vi "Actor Core.vi"(8 "error in":errorcluster, 11 "PS in":refnum<class "Power Supply.lvclass">) -> (0 "error out":errorcluster, 3 "Actor out":refnum<class "Actor.lvclass">)   [LabVIEW 2019, in "Power Supply.lvlib" / "Power Supply.lvclass"]
doc: "The user interface for this panel.\n\n----\nPlease see the following web address for additional documentation and tutorial information:\nhttp://www.mooregoodideas.com/mgi-panel-manager/\n\nAuthor: Derek Trepanier\n\nCopyright (c) 2018, Moore Good Ideas, Inc.\n\nAll rights reserved.\n\nRedistribution and use in source and binary forms, with or without modification, are permitted provided that the following conditions are met:\n\n * Redistributions of source code must retain the above copyright notice, this list of conditions and the following disclaimer.\n * Redistributions in binary form must reproduce the above copyright notice, this list of conditions and the following disclaimer in the documentation and/or other materials provided with the distribution.\n * Neither the name of Moore Good Ideas, Inc. nor the names of its contributors may be used to endorse or promote products derived from this software without specific prior written permission.\n\nTHIS SOFTWARE IS PROVIDED BY THE COPYRIGHT HOLDERS AND CONTRIBUTORS \"AS IS\" AND ANY EXPRESS OR IMPLIED WARRANTIES, INCLUDING, BUT NOT LIMITED TO, THE IMPLIED WARRANTIES OF MERCHANTABILITY AND FITNESS FOR A PARTICULAR PURPOSE ARE DISCLAIMED. IN NO EVENT SHALL THE COPYRIGHT OWNER OR CONTRIBUTORS BE LIABLE FOR ANY DIRECT, INDIRECT, INCIDENTAL, SPECIAL, EXEMPLARY, OR CONSEQUENTIAL DAMAGES (INCLUDING, BUT NOT LIMITED TO, PROCUREMENT OF SUBSTITUTE GOODS OR SERVICES; LOSS OF USE, DATA, OR PROFITS; OR BUSINESS INTERRUPTION) HOWEVER CAUSED AND ON ANY THEORY OF LIABILITY, WHETHER IN CONTRACT, STRICT LIABILITY, OR TORT (INCLUDING NEGLIGENCE OR OTHERWISE) ARISING IN ANY WAY OUT OF THE USE OF THIS SOFTWARE, EVEN IF ADVISED OF THE POSSIBILITY OF SUCH DAMAGE."
uses:
  Power Supply.lvclass
  <vilib>/ActorFramework/Actor/Actor.lvclass
  C:/Program Files (x86)/National Instruments/LabVIEW 2019/vi.lib/MGI/Panel Manager/Panel Actor/Panel Actor/Panel Actor.lvclass
  Power Supply.lvclass/Power Supply.ctl
  Serial/Serial Messages/Write Msg/Write Msg.lvclass/Write Msg.ctl
  <vilib>/ActorFramework/Message Enqueuer/Message Enqueuer.lvclass/Message Enqueuer.ctl
  Serial/Serial Messages/Read Msg/Read Msg.lvclass/Read Msg.ctl
  Serial/Serial Messages/Config Msg/Config Msg.lvclass/Config Msg.ctl
  <vilib>/ActorFramework/Message Enqueuer/Enqueue.vi
  Serial/Serial Messages/Write Msg/Write Msg.lvclass
  C:/Program Files (x86)/National Instruments/LabVIEW 2019/vi.lib/ActorFramework/Message/Message.lvclass
  Serial/Serial Messages/Read Msg/Read Msg.lvclass
  Serial/Serial Messages/Config Msg/Config Msg.lvclass
  Serial/Serial Messages/Close Msg/Close Msg.lvclass
  <vilib>/ActorFramework/Stop Msg/Stop Msg.lvclass
  <vilib>/ActorFramework/Message Priority Queue/Priority Enqueue.vi
  Instrument/Instrument/Instrument.lvclass
  <vilib>/MGI/Panel Manager/Panel Actor/Panel Actor/Panel Actor.lvclass
  Power Supply Messages/PS Dataset Msg/PS Dataset Msg.lvclass
  C:/Program Files (x86)/National Instruments/LabVIEW 2019/vi.lib/ActorFramework/Actor/Actor.lvclass
panel:
  in  "Simulation":bool
  out "Data":dbl[](array[numeric])
  in  "Serial Port":string(combo)="COM6" caption="Default Pattern Folder"
  in  "Baud rate":u32(ring)=19200 caption="Ring" items=["7200"=7200, "9600"=9600, "14400"=14400, "19200"=19200]
  out "Setpoint":dbl
  out "Output":bool
  out "Query":string
  out "Connected":bool
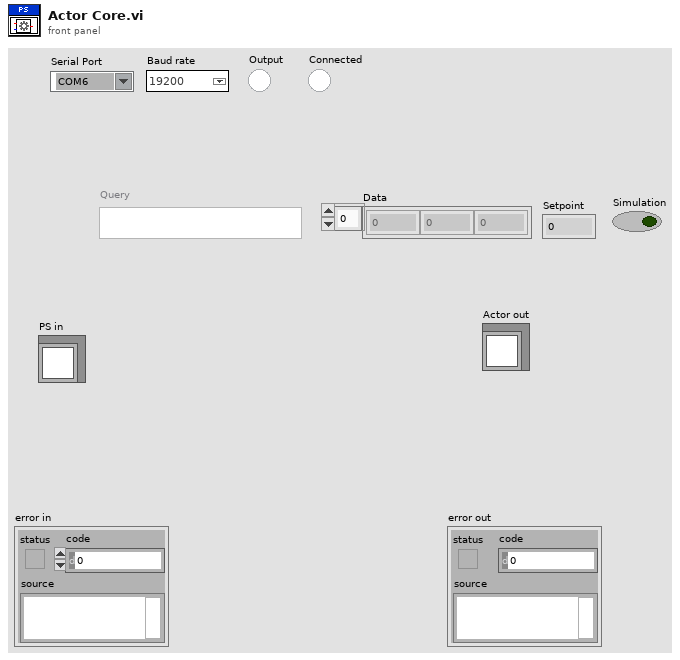
[diagram p1: front panel]
types:
  T1 = enum32{"Invalid", "Standard", "Closed", "Hidden", "Minimized", "Maximized"}
  T2 = cluster{"Event Registration Refnum":refnum<event-registration>, "Pnl Actor":refnum<event-registration>}
  T3 = enum8{"Enabled", "Disabled", "Disabled and Grayed Out"}
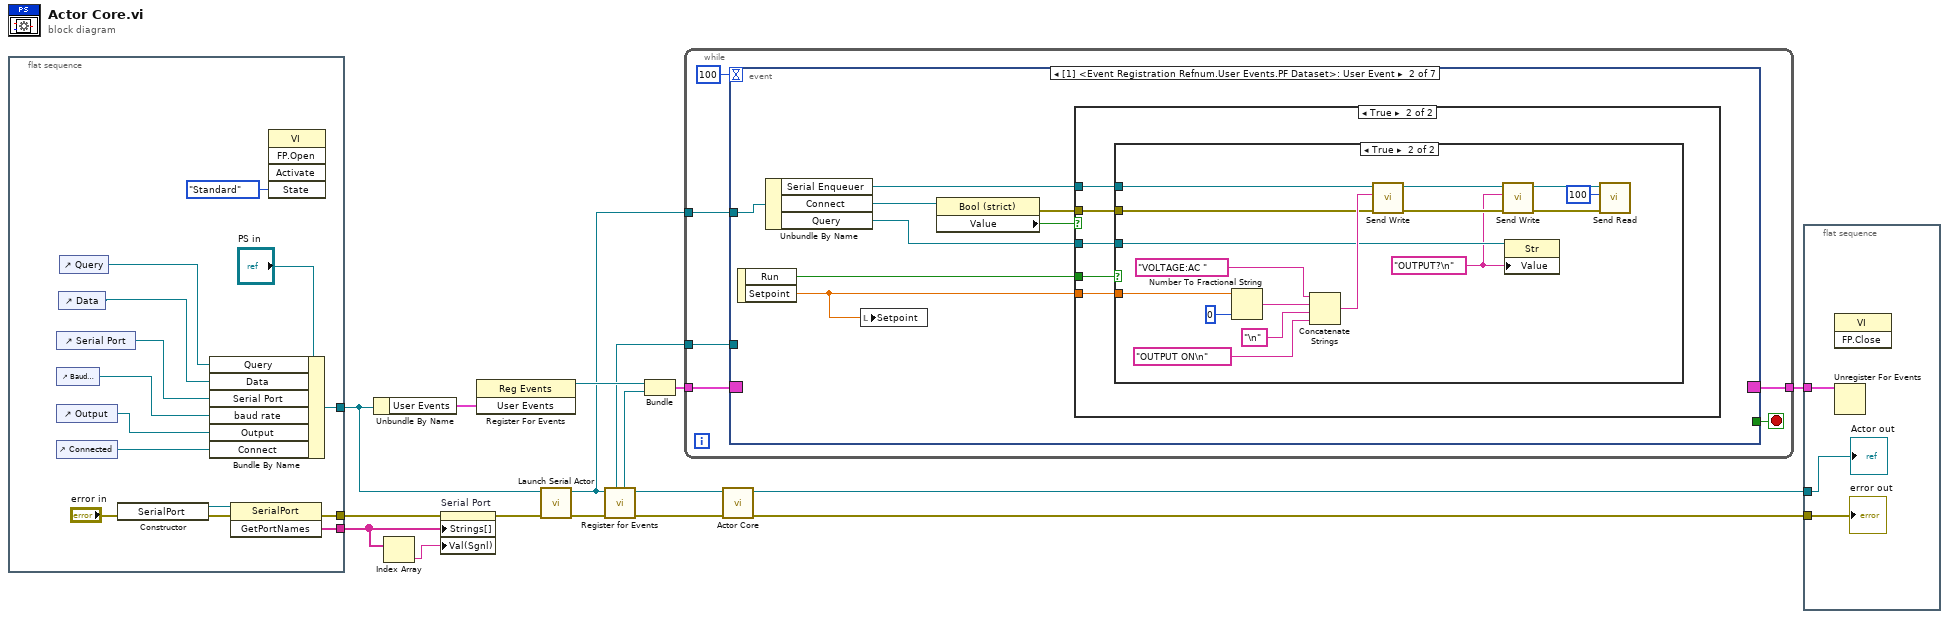
[diagram p0: block diagram]
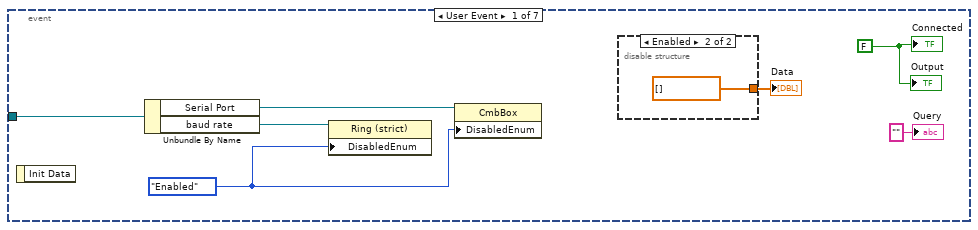
[diagram p2: hidden frame]
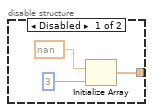
[diagram p3: hidden frame]
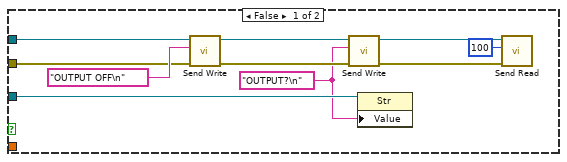
[diagram p5: hidden frame]
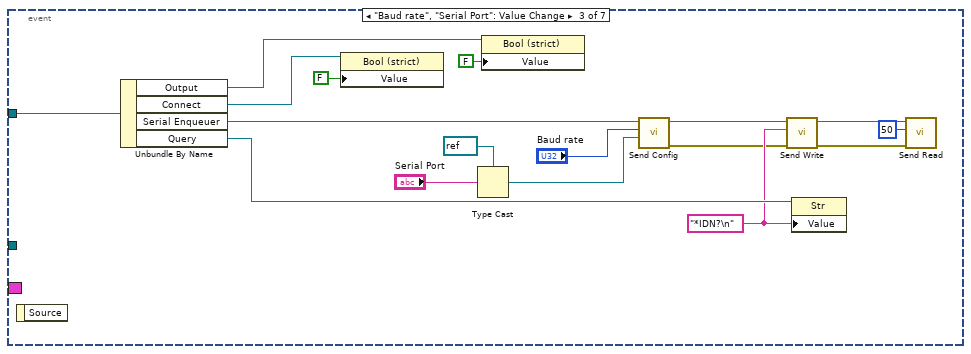
[diagram p6: hidden frame]
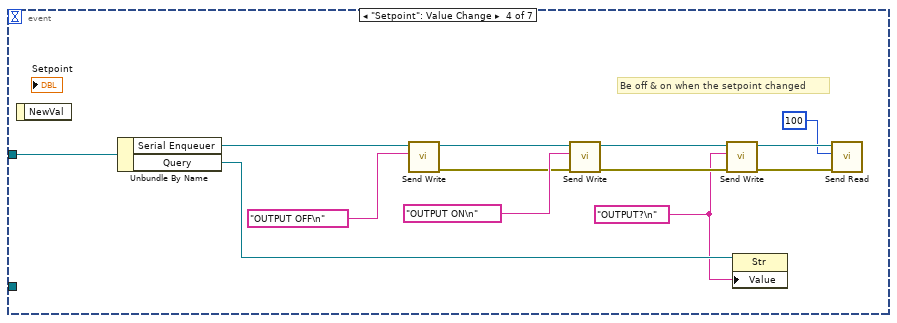
[diagram p7: hidden frame]
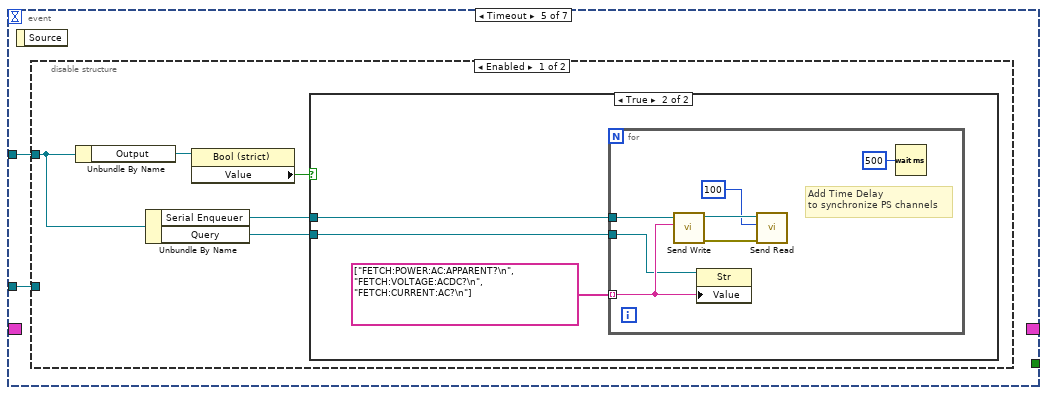
[diagram p8: hidden frame]
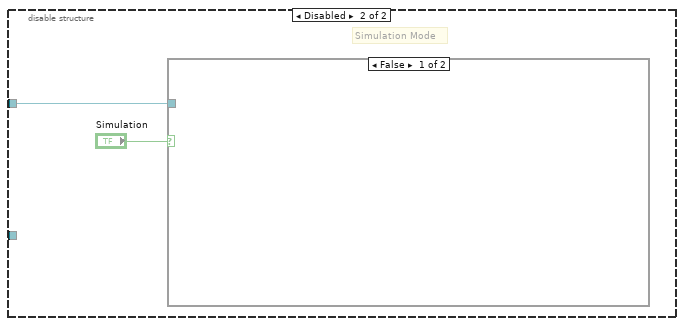
[diagram p10: hidden frame]
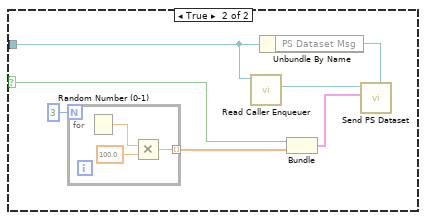
[diagram p11: hidden frame]
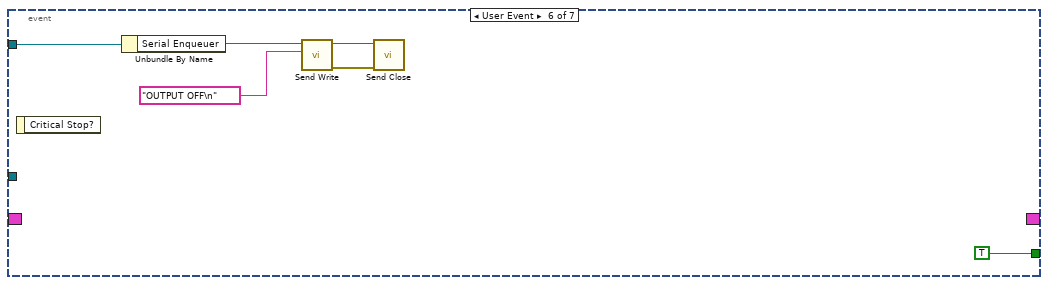
[diagram p12: hidden frame]
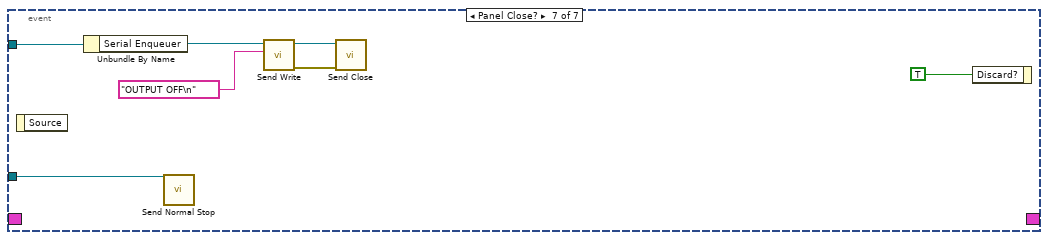
[diagram p13: hidden frame]
diagram:
  n1 = flat-sequence {
    tunnel: [w24] -> w7
    tunnel: [w29] -> w1
    tunnel: [w23] -> w5
    frame #0 {
      n2 = control-ref of="Serial Port"() -> (w20:refnum<vi>)
      n3 = control-ref of="Baud rate"() -> (w21:refnum<vi>)
      n4 = control-ref of="Output"() -> (w28:refnum<vi>)
      n5 = control-ref of="Connected"() -> (w30:refnum<vi>)
      n6 = control-ref of="Data"() -> (w19:refnum<vi>)
      n7 = control-ref of="Query"() -> (w18:refnum<vi>)
      n8 = constructor class="SerialPort"(error in="error in") -> (reference out=w26:refnum<k24>, error out=w27:errorcluster)  [unwired: 2 in, 1 out]
      n9 = Bundle By Name(cluster="PS in", "Query"=w18, "Data"=w19, "Serial Port"=w20, "baud rate"=w21, "Output"=w28, "Connect"=w30) -> (w29:refnum<class "Power Supply.lvclass">)
      n10 = invoke on="인보크 노드" class="SerialPort" method="GetPortNames"(reference=w26, error in=w27) -> (error out=w24:errorcluster, "GetPortNames"=w23:string[])  [unwired: 1 in, 1 out]
      n11 = invoke class="VI" method="FP.Open"("State"=T1."Standard") -> ()  [unwired: 4 in, 5 out]
    }
  }
  n12 = Unbundle By Name(w1) -> ("User Events"=w16:cluster{"PF Dataset":refnum<user-event>})
  n13 = Index Array(array=w5) -> (element=w4:string)  [unwired: 1 in]
  n14 = property on="Serial Port" class="CmbBox"(error in=w7, "Strings[]"=w5, "Val(Sgnl)"=w4) -> (error out=w6:errorcluster)  [unwired: 1 in, 1 out]
  n15 = register-events(w16) -> (reference out=w10:refnum<event-registration>)  [unwired: 2 in, 1 out]
  n16 = call "Launch Serial Actor.vi"("error in"=w6, "PS in"=w1) -> ("error out"=w8:errorcluster, "PS out"=w3:refnum<class "Power Supply.lvclass">)  [unwired: 8 in]
  n17 = call <vilib>:"Register for Events.vi"("Error In"=w8, "Panel Actor in"=w3) -> ("Error Out"=w13:errorcluster, "Panel Actor out"=w12:refnum<class "Power Supply.lvclass">, "Pnl Actor"=w11:refnum<event-registration>, "Self Enqueuer"=w9:refnum<class "Message Enqueuer.lvclass">)  [unwired: 6 in]
  n18 = Bundle("Event Registration Refnum"=w10, "Pnl Actor"=w11) -> (w15:T2)  [unwired: 1 in]
  n19 = while {
    tunnel: w15 -> [w37]
    tunnel: w9 -> [w36]
    tunnel: [w34] -> w14
    tunnel: w3 -> [w33]
    stop <- w35 stop-if-true
    n20 = event shown="[1] <Event Registration Refnum.User Events.PF Dataset>: User Event" {
      selector: w37 -> [_ _ _ _ _ _ _]
      dyn-events: [_ _ _ _ _ _ _] -> w34
      timeout: 100 -> [_ _ _ _ _ _ _]
      tunnel: w36 -> [_ _ _ _ w118 _ w158]
      tunnel: [_ _ _ _ _ TRUE _] -> w35
      tunnel: w33 -> [w39 w51 w104 w117 w119 w151 w153]
      event User Event {
        w40 = T3."Enabled" ("Disabled")
        w43 = FALSE ("Connect")
        n21 = event-data() -> ()  [unwired: 1 in, 1 out]
        n22 = Unbundle By Name(w39) -> ("Serial Port"=w41:refnum<vi>, "baud rate"=w42:refnum<vi>)
        n23 = property class="Ring (strict)"(reference=w42, "DisabledEnum"=w40) -> ()  [unwired: 1 in, 2 out]
        n24 = property class="CmbBox"(reference=w41, "DisabledEnum"=w40) -> ()  [unwired: 1 in, 2 out]
        n25 = disable-structure shown="Enabled" {
          disable-tunnel: [w46 dbl[] [] ("Data")] -> w44
          frame Disabled {
            n26 = Initialize Array(nan, 3 ("dimension size")) -> (w46:dbl[])
          }
          frame Enabled {
          }
        }
        "Data" <- w44
        "Connected" <- w43
        "Output" <- w43
        "Query" <- "" ("Query")
      }
      event User Event {
        n27 = event-data() -> ("Run"=w56:bool, "Setpoint"=w55:dbl)  [unwired: 1 in]
        n28 = Unbundle By Name(w51) -> ("Serial Enqueuer"=w54:refnum<class "Message Enqueuer.lvclass">, "Connect"=w52:refnum<vi>, "Query"=w50:refnum<vi>)
        n29 = local write "Setpoint"(w55) -> ()
        n30 = property class="Bool (strict)"(reference=w52) -> (error out=w49:errorcluster, "Value"=w53:bool)  [unwired: 1 in, 1 out]
        n31 = case shown="True" w53 {
          tunnel: w56 -> [_ w61]
          tunnel: w55 -> [_ w60]
          tunnel: w54 -> [_ w59]
          tunnel: w50 -> [_ w58]
          tunnel: w49 -> [_ w57]
          frame False {
          }
          frame True {
            n32 = case shown="True" w61 {
              tunnel: w59 -> [w71 w87]
              tunnel: w60 -> [_ w86]
              tunnel: w58 -> [w67 w77]
              tunnel: w57 -> [w63 w75]
              frame False {
                w64 = "OUTPUT?\n" ("Command")
                n33 = call "Send Write.vi"("error in (no error)"=w63, "Command"="OUTPUT OFF\n", "Message Enqueuer"=w71) -> ("error out"=w70:errorcluster, "Message Enqueuer out"=w69:refnum<class "Message Enqueuer.lvclass">)  [unwired: 7 in]
                n34 = call "Send Write.vi"("error in (no error)"=w70, "Command"=w64, "Message Enqueuer"=w69) -> ("error out"=w66:errorcluster, "Message Enqueuer out"=w65:refnum<class "Message Enqueuer.lvclass">)  [unwired: 7 in]
                n35 = property class="Str"(reference=w67, "Value"=w64) -> ()  [unwired: 1 in, 2 out]
                n36 = call "Send Read.vi"("error in (no error)"=w66, "delay before read (100ms)"=u32 100, "Message Enqueuer"=w65) -> ()  [unwired: 7 in, 2 out]
              }
              frame True {
                w76 = "OUTPUT?\n" ("Command")
                n37 = Number To Fractional String(number=w86, precision (6)=0) -> (F-format string=w85:string)  [unwired: 1 in, 1 out]
                n38 = Concatenate Strings("VOLTAGE:AC " ("Command"), w85, "\n" ("Command"), "OUTPUT ON\n" ("Command")) -> (w84:string)
                n39 = call "Send Write.vi"("error in (no error)"=w75, "Command"=w84, "Message Enqueuer"=w87) -> ("error out"=w78:errorcluster, "Message Enqueuer out"=w79:refnum<class "Message Enqueuer.lvclass">)  [unwired: 7 in]
                n40 = call "Send Write.vi"("error in (no error)"=w78, "Command"=w76, "Message Enqueuer"=w79) -> ("error out"=w74:errorcluster, "Message Enqueuer out"=w73:refnum<class "Message Enqueuer.lvclass">)  [unwired: 7 in]
                n41 = property class="Str"(reference=w77, "Value"=w76) -> ()  [unwired: 1 in, 2 out]
                n42 = call "Send Read.vi"("error in (no error)"=w74, "delay before read (100ms)"=u32 100, "Message Enqueuer"=w73) -> ()  [unwired: 7 in, 2 out]
              }
            }
          }
        }
      }
      event "Baud rate", "Serial Port": Value Change {
        w94 = "*IDN?\n" ("Command")
        n43 = event-data() -> ()  [unwired: 1 in, 1 out]
        n44 = Unbundle By Name(w104) -> ("Output"=w93:refnum<vi>, "Connect"=w97:refnum<vi>, "Serial Enqueuer"=w103:refnum<class "Message Enqueuer.lvclass">, "Query"=w95:refnum<vi>)
        n45 = property class="Bool (strict)"(reference=w97, "Value"=FALSE) -> ()  [unwired: 1 in, 2 out]
        n46 = Type Cast(type=refnum<visa-resource-name> refnum ("VISA resource name"), x="Serial Port") -> (*(type *) &x=w100:refnum<visa-resource-name>)
        n47 = property class="Bool (strict)"(reference=w93, "Value"=FALSE) -> ()  [unwired: 1 in, 2 out]
        n48 = call "Send Config.vi"("VISA resource name"=w100, "baud rate"="Baud rate", "Message Enqueuer"=w103) -> ("error out"=w91:errorcluster, "Message Enqueuer out"=w99:refnum<class "Message Enqueuer.lvclass">)  [unwired: 7 in]
        n49 = call "Send Write.vi"("error in (no error)"=w91, "Command"=w94, "Message Enqueuer"=w99) -> ("error out"=w90:errorcluster, "Message Enqueuer out"=w89:refnum<class "Message Enqueuer.lvclass">)  [unwired: 7 in]
        n50 = property class="Str"(reference=w95, "Value"=w94) -> ()  [unwired: 1 in, 2 out]
        n51 = call "Send Read.vi"("error in (no error)"=w90, "delay before read (100ms)"=u32 50, "Message Enqueuer"=w89) -> ()  [unwired: 7 in, 2 out]
      }
      event "Setpoint": Value Change {
        w106 = "OUTPUT?\n" ("Command")
        # "Be off & on when the setpoint changed"
        n52 = event-data() -> ()  [unwired: 1 in, 1 out]
        n53 = Unbundle By Name(w117) -> ("Serial Enqueuer"=w116:refnum<class "Message Enqueuer.lvclass">, "Query"=w107:refnum<vi>)
        n54 = call "Send Write.vi"("Command"="OUTPUT OFF\n", "Message Enqueuer"=w116) -> ("error out"=w109:errorcluster, "Message Enqueuer out"=w108:refnum<class "Message Enqueuer.lvclass">)  [unwired: 8 in]
        n55 = call "Send Write.vi"("error in (no error)"=w109, "Command"="OUTPUT ON\n", "Message Enqueuer"=w108) -> ("error out"=w112:errorcluster, "Message Enqueuer out"=w111:refnum<class "Message Enqueuer.lvclass">)  [unwired: 7 in]
        n56 = call "Send Write.vi"("error in (no error)"=w112, "Command"=w106, "Message Enqueuer"=w111) -> ("error out"=w114:errorcluster, "Message Enqueuer out"=w113:refnum<class "Message Enqueuer.lvclass">)  [unwired: 7 in]
        n57 = property class="Str"(reference=w107, "Value"=w106) -> ()  [unwired: 1 in, 2 out]
        n58 = call "Send Read.vi"("error in (no error)"=w114, "delay before read (100ms)"=u32 100, "Message Enqueuer"=w113) -> ()  [unwired: 7 in, 2 out]
      }
      event Timeout {
        n59 = event-data() -> ()  [unwired: 1 in, 1 out]
        n60 = disable-structure shown="Enabled" {
          disable-tunnel: w119 -> [w122 w136]
          disable-tunnel: w118 -> [_ _]
          frame Enabled {
            n61 = Unbundle By Name(w122) -> ("Output"=w124:refnum<vi>)
            n62 = Unbundle By Name(w122) -> ("Serial Enqueuer"=w121:refnum<class "Message Enqueuer.lvclass">, "Query"=w120:refnum<vi>)
            n63 = property class="Bool (strict)"(reference=w124) -> ("Value"=w123:bool)  [unwired: 1 in, 2 out]
            n64 = case shown="True" w123 {
              tunnel: w121 -> [_ w127]
              tunnel: w120 -> [_ w126]
              frame False {
              }
              frame True {
                n65 = for {
                  tunnel: string[] ["FETCH:POWER:AC:APPARENT?\n", "FETCH:VOLTAGE:ACDC?\n", "FETCH:CURRENT:AC?\n"] -> [w132] mode=indexing
                  tunnel: w127 -> [w130]
                  tunnel: w126 -> [w129]
                  # "Add Time Delay\nto synchronize PS channels"
                  n66 = call "Send Write.vi"("Command"=w132, "Message Enqueuer"=w130) -> ("error out"=w133:errorcluster, "Message Enqueuer out"=w134:refnum<class "Message Enqueuer.lvclass">)  [unwired: 8 in]
                  n67 = property class="Str"(reference=w129, "Value"=w132) -> ()  [unwired: 1 in, 2 out]
                  n68 = call "Send Read.vi"("error in (no error)"=w133, "delay before read (100ms)"=u32 100, "Message Enqueuer"=w134) -> ()  [unwired: 7 in, 2 out]
                  n69 = Wait (ms)(milliseconds to wait=u32 500) -> ()  [unwired: 1 out]
                }
              }
            }
          }
          frame Disabled {
            # "Simulation Mode"
            n70 = case shown="False" "Simulation" {
              selector: "Simulation" -> [_ w142]
              tunnel: w136 -> [_ w143]
              frame False {
              }
              frame True {
                n71 = for {
                  N: 3 -> [_]
                  tunnel: [w144] -> w140 mode=indexing
                  n72 = Random Number (0-1)() -> (number: 0 to 1=w145:dbl)
                  n73 = Multiply(x=w145, y=100.0) -> (x*y=w144:dbl)
                }
                n74 = call <vilib>:"Read Caller Enqueuer.vi"("Actor"=w143) -> ("Caller Enqueuer"=w138:refnum<class "Message Enqueuer.lvclass">)  [unwired: 10 in]
                n75 = Unbundle By Name(w143) -> ("PS Dataset Msg"=w139:refnum<class "PS Dataset Msg.lvclass">)
                n76 = Bundle(w142, w140) -> (w137:cluster{bool, dbl[]})  [unwired: 1 in]
                n77 = call "Send PS Dataset.vi"("Message Type"=w139, "PS Dataset"=w137, "Message Enqueuer"=w138) -> ()  [unwired: 7 in, 2 out]
              }
            }
          }
        }
      }
      event User Event {
        n78 = event-data() -> ()  [unwired: 1 in, 1 out]
        n79 = Unbundle By Name(w151) -> ("Serial Enqueuer"=w148:refnum<class "Message Enqueuer.lvclass">)
        n80 = call "Send Write.vi"("Command"="OUTPUT OFF\n", "Message Enqueuer"=w148) -> ("error out"=w150:errorcluster, "Message Enqueuer out"=w149:refnum<class "Message Enqueuer.lvclass">)  [unwired: 8 in]
        n81 = call "Send Close.vi"("error in (no error)"=w150, "Message Enqueuer"=w149) -> ()  [unwired: 8 in, 2 out]
      }
      event Panel Close? {
        n82 = event-data() -> ()  [unwired: 1 in, 1 out]
        n83 = Unbundle By Name(w153) -> ("Serial Enqueuer"=w155:refnum<class "Message Enqueuer.lvclass">)
        n84 = call <vilib>:"Send Normal Stop.vi"("Message Enqueuer"=w158) -> ()  [unwired: 10 in, 1 out]
        n85 = call "Send Write.vi"("Command"="OUTPUT OFF\n", "Message Enqueuer"=w155) -> ("error out"=w157:errorcluster, "Message Enqueuer out"=w156:refnum<class "Message Enqueuer.lvclass">)  [unwired: 8 in]
        n86 = call "Send Close.vi"("error in (no error)"=w157, "Message Enqueuer"=w156) -> ()  [unwired: 8 in, 2 out]
        n87 = event-data("Discard?"=TRUE) -> ()  [unwired: 1 in, 1 out]
      }
    }
  }
  n88 = call-parent "Actor Core.vi"("error in"=w13, "Instrument in"=w12) -> ("error out"=w17:errorcluster, "Actor out"=w2:refnum<class "Actor.lvclass">)  [unwired: 8 in]
  n89 = flat-sequence {
    tunnel: w17 -> [w162]
    tunnel: w2 -> [w160]
    tunnel: w14 -> [w161]
    frame #0 {
      n90 = invoke class="VI" method="FP.Close"() -> ()  [unwired: 3 in, 3 out]
      n91 = Unregister For Events(event registration refnum=w161) -> ()  [unwired: 1 in, 1 out]
      "error out" <- w162
      "Actor out" <- w160
    }
  }
